vi "projectpathsubvi.vi"() -> (3 "stripped path":path)   [LabVIEW 2018, in "analysis.lvlib"]
uses:
  analysis.lvlib
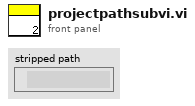
[diagram p1: front panel]
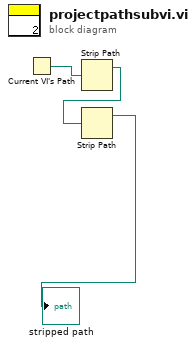
[diagram p0: block diagram]
diagram:
  n1 = Current VI's Path() -> (path=w1:path)
  n2 = Strip Path(path=w1) -> (stripped path=w2:path)  [unwired: 1 out]
  n3 = Strip Path(path=w2) -> (stripped path=→"stripped path":path)  [unwired: 1 out]
